vi "get_ID.vi"(8 "error in (no error)":errorcluster, 11 "Simulated_Instrument in":refnum<class "Simulated_Instrument.lvclass">) -> (0 "error out":errorcluster, 2 "ID from Instrument":string, 3 "Simulated_Instrument out":refnum<class "Simulated_Instrument.lvclass">)   [LabVIEW 2017, in "Simulated_Instrument.lvclass"]
doc: "the vi reads the ID from the instrument"
uses:
  Simulated_Instrument.lvclass
  instrument.lvclass
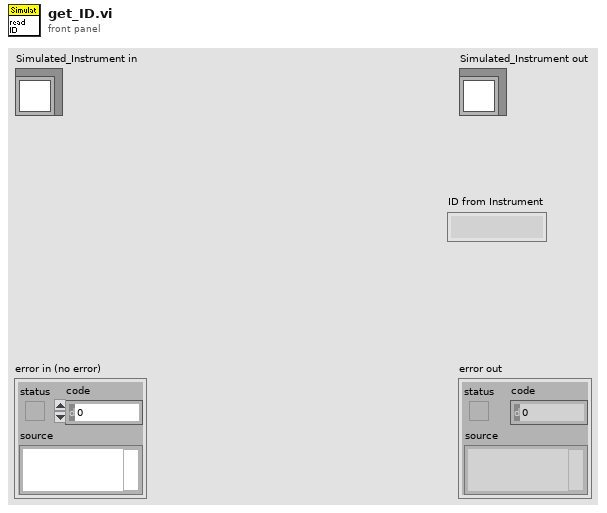
[diagram p1: front panel]
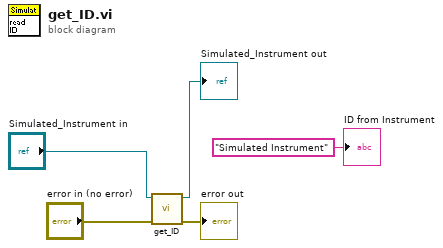
[diagram p0: block diagram]
diagram:
  n1 = call-parent "get_ID.vi"("error in (no error)"="error in (no error)", "instrument in"="Simulated_Instrument in") -> ("error out"=→"error out":errorcluster, "instrument out"=→"Simulated_Instrument out":refnum<class "Simulated_Instrument.lvclass">)  [unwired: 7 in, 1 out]
  "ID from Instrument" <- "Simulated Instrument" ("ID from Instrument")
